vi "Note Result.vi"(8 "error in (no error)":errorcluster, 9 "Stage":enum16{"Init", "Work"}(ring), 10 "Acquired Result.lvclass":refnum<class "Acquired Result.lvclass">, 11 "Measure Controller in":refnum<class "Process Controller.lvclass">) -> (0 "error out":errorcluster, 2 "Awaiting results":bool, 3 "Measure Controller out":refnum<class "Process Controller.lvclass">)   [LabVIEW 2021, in "Process Controller.lvclass"]
uses:
  Process Controller.lvclass
  NHMFL_Core/Libraries/Instruments/Results/Acquired Result/Acquired Result.lvclass
  NHMFL_Core/Libraries/Instruments/Results/Acquired Result/Acquired Result.lvclass/Acquired Result.ctl
  Process Controller.lvclass/Process Controller.ctl
  NHMFL_Core/Libraries/Instruments/Results/Acquired Result/Read Sender.vi
  NHMFL_Core/Libraries/Instruments/Results/Acquired Result/Read Final.vi
  NHMFL_Core/Libraries/Instruments/Results/Acquired Result/Read Cycle count.vi
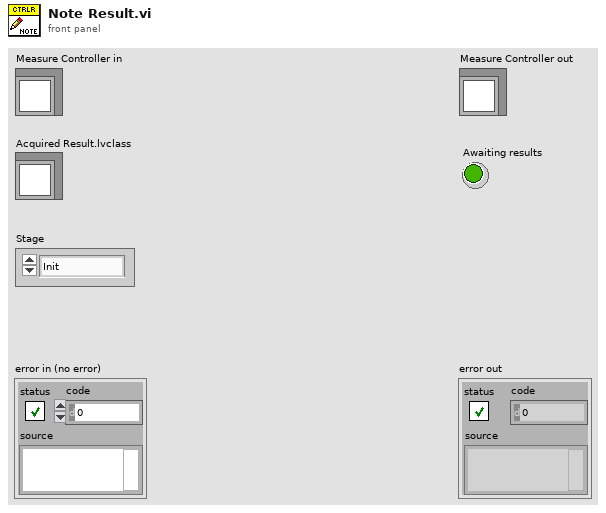
[diagram p1: front panel]
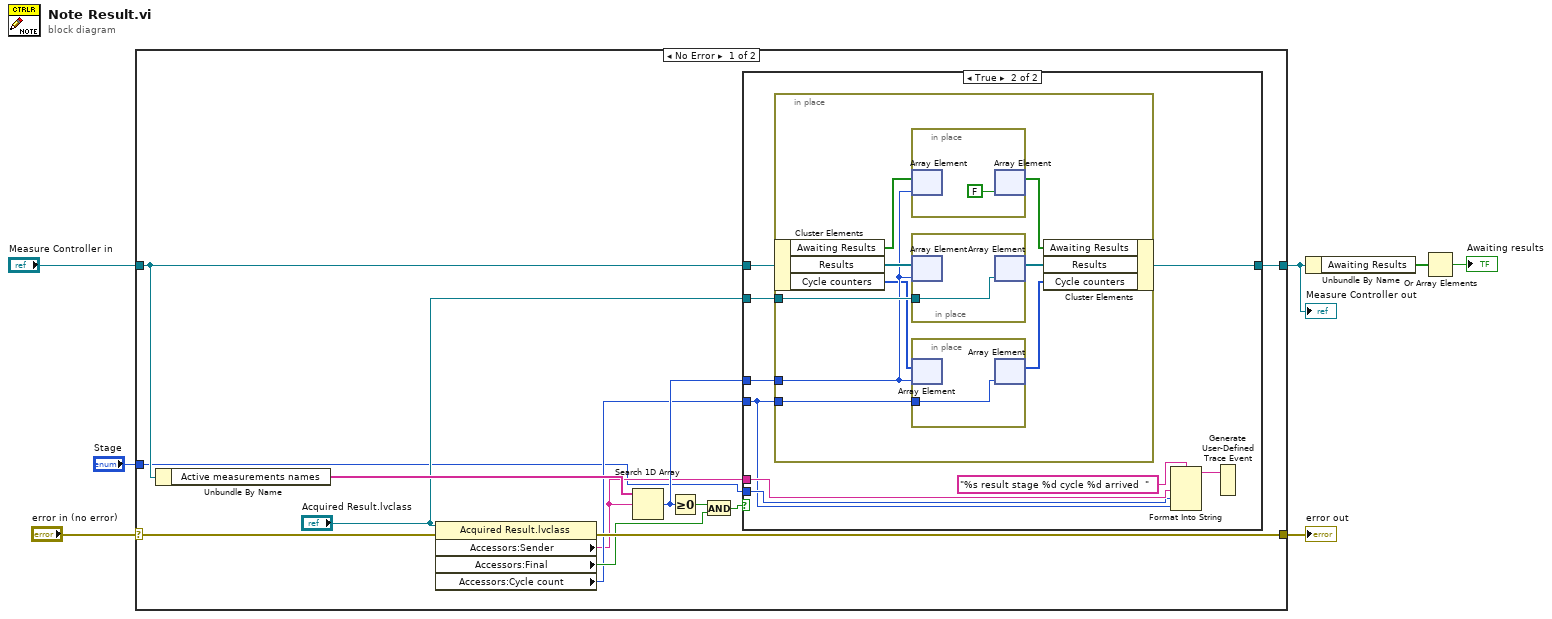
[diagram p0: block diagram]
diagram:
  n1 = case shown="No Error" "error in (no error)" {
    selector: "error in (no error)" -> [w18 w44]
    tunnel: [w17 w44] -> w6
    tunnel: [w15 w43] -> w3
    tunnel: "Measure Controller in" -> [w16 w43]
    tunnel: "Stage" -> [w8 _]
    frame No Error {
      n2 = Unbundle By Name(w16) -> ("Active measurements names"=w20:string[])
      n3 = property class="Acquired Result.lvclass"(reference="Acquired Result.lvclass", error in=w18) -> (error out=w17:errorcluster, "Accessors:Sender"=w9:string, "Accessors:Final"=w11:bool, "Accessors:Cycle count"=w10:i32)  [unwired: 1 out]
      n4 = Search 1D Array(1D array=w20, element=w9) -> (index of element=w13:i32)  [unwired: 1 in]
      n5 = Greater Or Equal To 0?(x=w13) -> (x >= 0?=w14:bool)
      n6 = And(x=w14, y=w11) -> (x .and. y?=w12:bool)
      n7 = case shown="True" w12 {
        tunnel: w13 -> [_ w30]
        tunnel: "Acquired Result.lvclass" -> [_ w29]
        tunnel: w16 -> [w21 w28]
        tunnel: [w21 w27] -> w15
        tunnel: w10 -> [_ w23]
        tunnel: w9 -> [_ w25]
        tunnel: w8 -> [_ w24]
        frame False {
        }
        frame True {
          n8 = in-place {
            in-place-border: w30 -> [w35]
            in-place-border: w29 -> [w37]
            in-place-border: w23 -> [w34]
            n9 = in-place-cluster #1(w28) -> ("Awaiting Results"=w39:bool[], "Results"=w38:refnum<class "Acquired Result.lvclass">[], "Cycle counters"=w33:i32[])
            n10 = in-place {
              n11 = in-place-array #2(w39, w35) -> ()  [unwired: 1 out]
              n12 = in-place-array #2(FALSE ("new element/subarray")) -> (w31:bool[])  [unwired: 1 out]
            }
            n13 = in-place {
              in-place-border: w37 -> [w41]
              n14 = in-place-array #3(w38, w35) -> ()  [unwired: 1 out]
              n15 = in-place-array #3(w41) -> (w36:refnum<class "Acquired Result.lvclass">[])  [unwired: 1 out]
            }
            n16 = in-place {
              in-place-border: w34 -> [w40]
              n17 = in-place-array #4(w33, w35) -> ()  [unwired: 1 out]
              n18 = in-place-array #4(w40) -> (w32:i32[])  [unwired: 1 out]
            }
            n19 = in-place-cluster #1("Awaiting Results"=w31, "Results"=w36, "Cycle counters"=w32) -> (w27:refnum<class "Process Controller.lvclass">)
          }
          n20 = Format Into String(format string="%s result stage %d cycle %d arrived  ", w25, w24, w23) -> (resulting string=w22:string)  [unwired: 2 in, 1 out]
          n21 = Generate User-Defined Trace Event(2:w22) -> ()  [unwired: 1 in]
        }
      }
    }
    frame Error {
    }
  }
  "error out" <- w6
  "Measure Controller out" <- w3
  n22 = Unbundle By Name(w3) -> ("Awaiting Results"=w1:bool[])
  n23 = Or Array Elements(Boolean array=w1) -> (logical OR=→"Awaiting results":bool)
